vi "Test - Add  Property (Boolean).vi"() -> ()   [LabVIEW 2020, in "JSON Schema Generator.lvlib"]
uses:
  JSON Schema Generator.lvlib
  <vilib>/addons/_JKI Toolkits/Caraya/classes/Test/Test.lvclass
  <vilib>/addons/_JKI Toolkits/Caraya/classes/Assert/Assert.lvclass
  <vilib>/JDP Science/JSONtext/JSONtext.lvlib
  <vilib>/addons/_JKI Toolkits/Caraya/classes/Assert/Assert Not Error.vi
  <vilib>/addons/_JKI Toolkits/Caraya/classes/Assert/Assert Equal Value_Variant.vi
panel:
  in  "New Boolean":bool
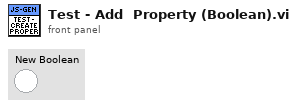
[diagram p1: front panel]
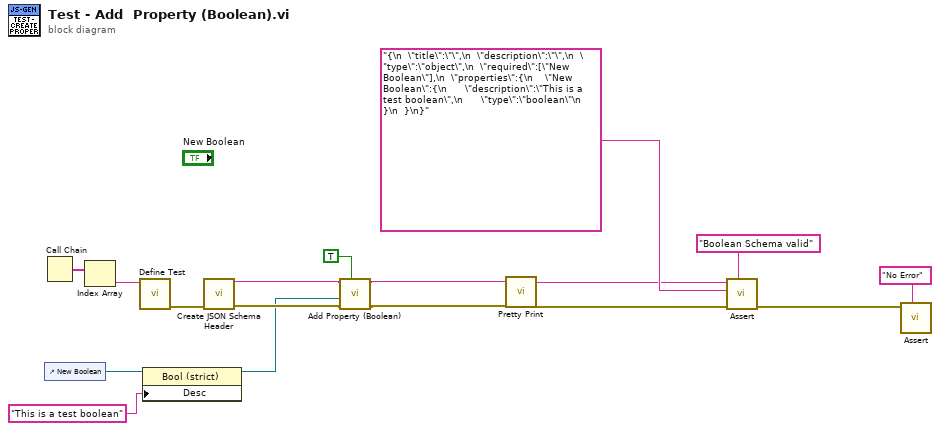
[diagram p0: block diagram]
diagram:
  n1 = Call Chain() -> (call chain=w17:string[])
  n2 = control-ref of="New Boolean"() -> (w5:refnum<vi>)
  n3 = Index Array(array=w17) -> (element=w16:string)  [unwired: 1 in]
  n4 = call <vilib>:"Define Test.vi"("Label (VI Title)"=w16) -> ("error out"=w12:errorcluster)  [unwired: 9 in, 1 out]
  n5 = property class="Bool (strict)"(reference=w5, "Desc"="This is a test boolean" ("Description")) -> (reference out=w3:refnum<vi>)  [unwired: 1 in, 1 out]
  n6 = call "Create JSON Schema Header.vi"("error in (no error)"=w12) -> ("error out"=w6:errorcluster, "JSON Schema out"=w9:string)  [unwired: 9 in]
  n7 = call "Add Property (Boolean).vi"("Required?"=TRUE, "error in (no error)"=w6, "String In"=w3, "JSON Schema in"=w9) -> ("error out"=w4:errorcluster, "JSON SChema out"=w8:string)  [unwired: 6 in]
  n8 = call <vilib>:"Pretty Print.vi"("error in (no error)"=w4, "JSON"=w8) -> ("error out"=w11:errorcluster, "<JSON>"=w1:string)  [unwired: 7 in, 1 out]
  n9 = call-poly <vilib>:"Assert.vi"("Label"="Boolean Schema valid", "error in (no error)"=w11, "Actual"="{\n  \"title\":\"\",\n  \"description\":\"\",\n  \"type\":\"object\",\n  \"required\":[\"New Boolean\"],\n  \"properties\":{\n    \"New Boolean\":{\n      \"description\":\"This is a test boolean\",\n      \"type\":\"boolean\"\n    }\n  }\n}", "Expected"=w1) -> ("error out"=w14:errorcluster)  [unwired: 6 in, 1 out]
  n10 = call-poly <vilib>:"Assert.vi"("Label"="No Error", "Not Error?"=w14) -> ()  [unwired: 8 in, 2 out]
